vi "Add Build Recipe.vi"(8 "error in (no error)":errorcluster, 10 "Build Recipe":refnum<class "Build Job.lvclass">[](array[class]), 11 "CI Project in":refnum<class "CI Project.lvclass">) -> (0 "error out":errorcluster, 3 "CI Project out":refnum<class "CI Project.lvclass">)   [LabVIEW 2014, in "CI Project.lvclass"]
uses:
  CI Project.lvclass
  Build Job/Build Job.lvclass
  CI Project.lvclass/CI Project.ctl
  Build Job/Build Job.lvclass/Build Job.ctl
  Build Job/Read Parameters.vi
  Build Job/Write Parameters.vi
  Build Job/Write Hostname.vi
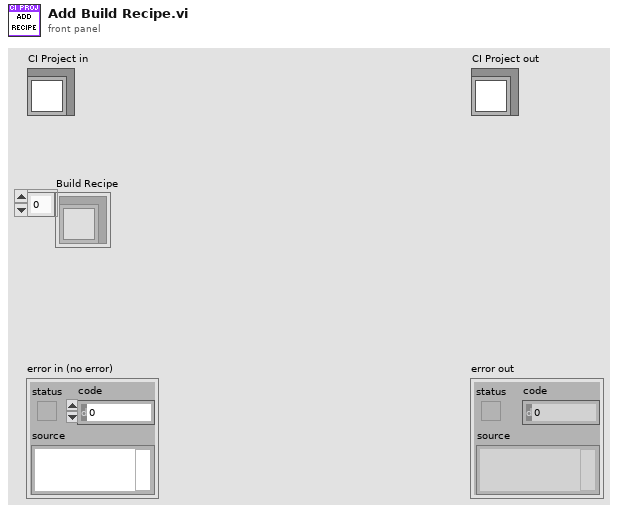
[diagram p1: front panel]
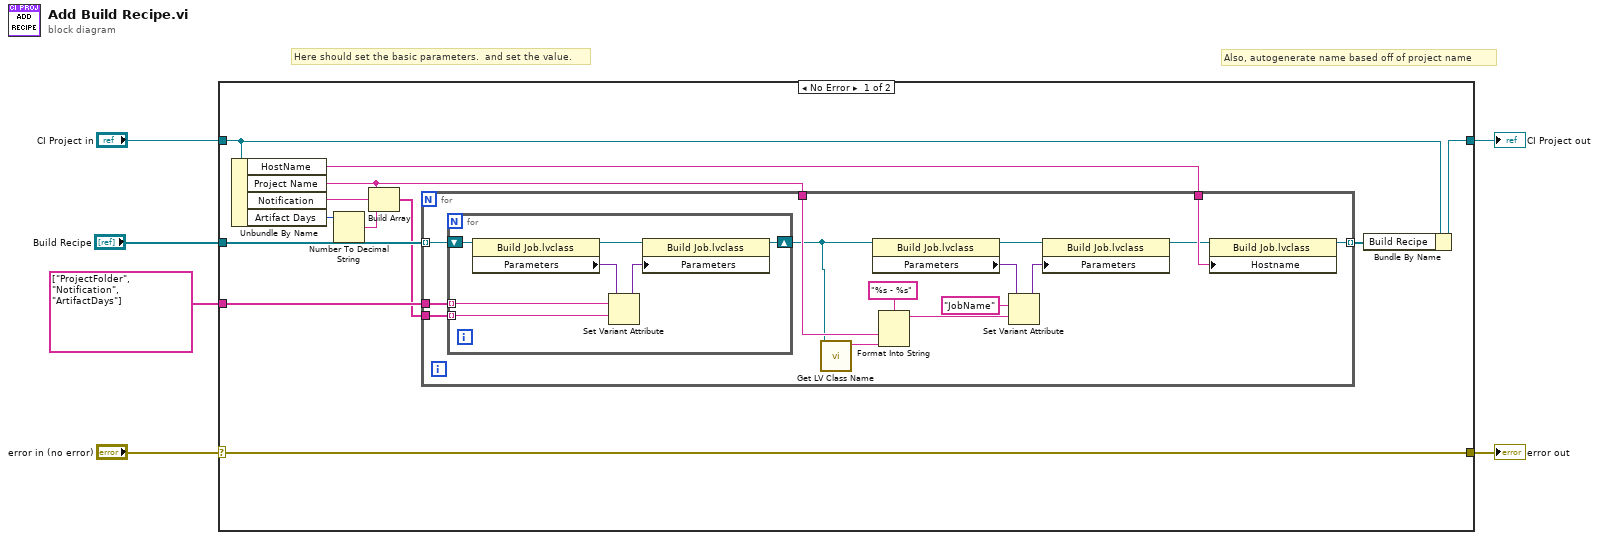
[diagram p0: block diagram]
diagram:
  # "Also, autogenerate name based off of project name"
  # "Here should set the basic parameters.  and set the value."
  n1 = case shown="No Error" "error in (no error)" {
    selector: "error in (no error)" -> [w18 w42]
    tunnel: [w18 w42] -> w5
    tunnel: [w17 w41] -> w3
    tunnel: "CI Project in" -> [w16 w41]
    tunnel: "Build Recipe" -> [w15 _]
    tunnel: string[] ["ProjectFolder", "Notification", "ArtifactDays"] -> [w13 _]
    frame No Error {
      n2 = Unbundle By Name(w16) -> ("HostName"=w10:string, "Project Name"=w9:string, "Notification"=w12:string, "Artifact Days"=w8:i32)
      n3 = Number To Decimal String(number=w8) -> (decimal integer string=w7:string)  [unwired: 1 in]
      n4 = Build Array(w9, w12, w7) -> (w11:string[])
      n5 = for {
        tunnel: w15 -> [w33] mode=indexing
        tunnel: [w29] -> w14 mode=indexing
        tunnel: w13 -> [w32]
        tunnel: w11 -> [w31]
        tunnel: w10 -> [w30]
        tunnel: w9 -> [w27]
        n6 = for {
          shift-right: [w40] -> w20
          shift-left: w33 -> [w39]
          tunnel: w32 -> [w35] mode=indexing
          tunnel: w31 -> [w34] mode=indexing
          n7 = property class="Build Job.lvclass"(reference=w39) -> (reference out=w38:refnum<class "Build Job.lvclass">, "Parameters"=w37:variant)  [unwired: 1 in, 1 out]
          n8 = Set Variant Attribute(Variant=w37, name=w35, value=w34) -> (Variant out=w36:variant)  [unwired: 1 in, 2 out]
          n9 = property class="Build Job.lvclass"(reference=w38, "Parameters"=w36) -> (reference out=w40:refnum<class "Build Job.lvclass">)  [unwired: 1 in, 1 out]
        }
        n10 = call <vilib>:"Get LV Class Name.vi"("object"=w20) -> ("class name"=w19:string)  [unwired: 9 in, 1 out]
        n11 = property class="Build Job.lvclass"(reference=w20) -> (reference out=w26:refnum<class "Build Job.lvclass">, "Parameters"=w25:variant)  [unwired: 1 in, 1 out]
        n12 = Format Into String(format string="%s - %s", w27, w19) -> (resulting string=w21:string)  [unwired: 2 in, 1 out]
        n13 = Set Variant Attribute(Variant=w25, name="JobName", value=w21) -> (Variant out=w24:variant)  [unwired: 1 in, 2 out]
        n14 = property class="Build Job.lvclass"(reference=w26, "Parameters"=w24) -> (reference out=w28:refnum<class "Build Job.lvclass">)  [unwired: 1 in, 1 out]
        n15 = property class="Build Job.lvclass"(reference=w28, "Hostname"=w30) -> (reference out=w29:refnum<class "Build Job.lvclass">)  [unwired: 1 in, 1 out]
      }
      n16 = Bundle By Name(cluster=w16, "Build Recipe"=w14) -> (w17:refnum<class "CI Project.lvclass">)
    }
    frame Error {
    }
  }
  "error out" <- w5
  "CI Project out" <- w3
